vi "VS Async VI_Example.vi"() -> ()   [LabVIEW 2011]
uses:
  CANOpen Addon Custom Device.lvlib
panel:
  in  "stop":bool
  in  "Error":errorcluster
  out "error out":errorcluster
  in  "Parent":string
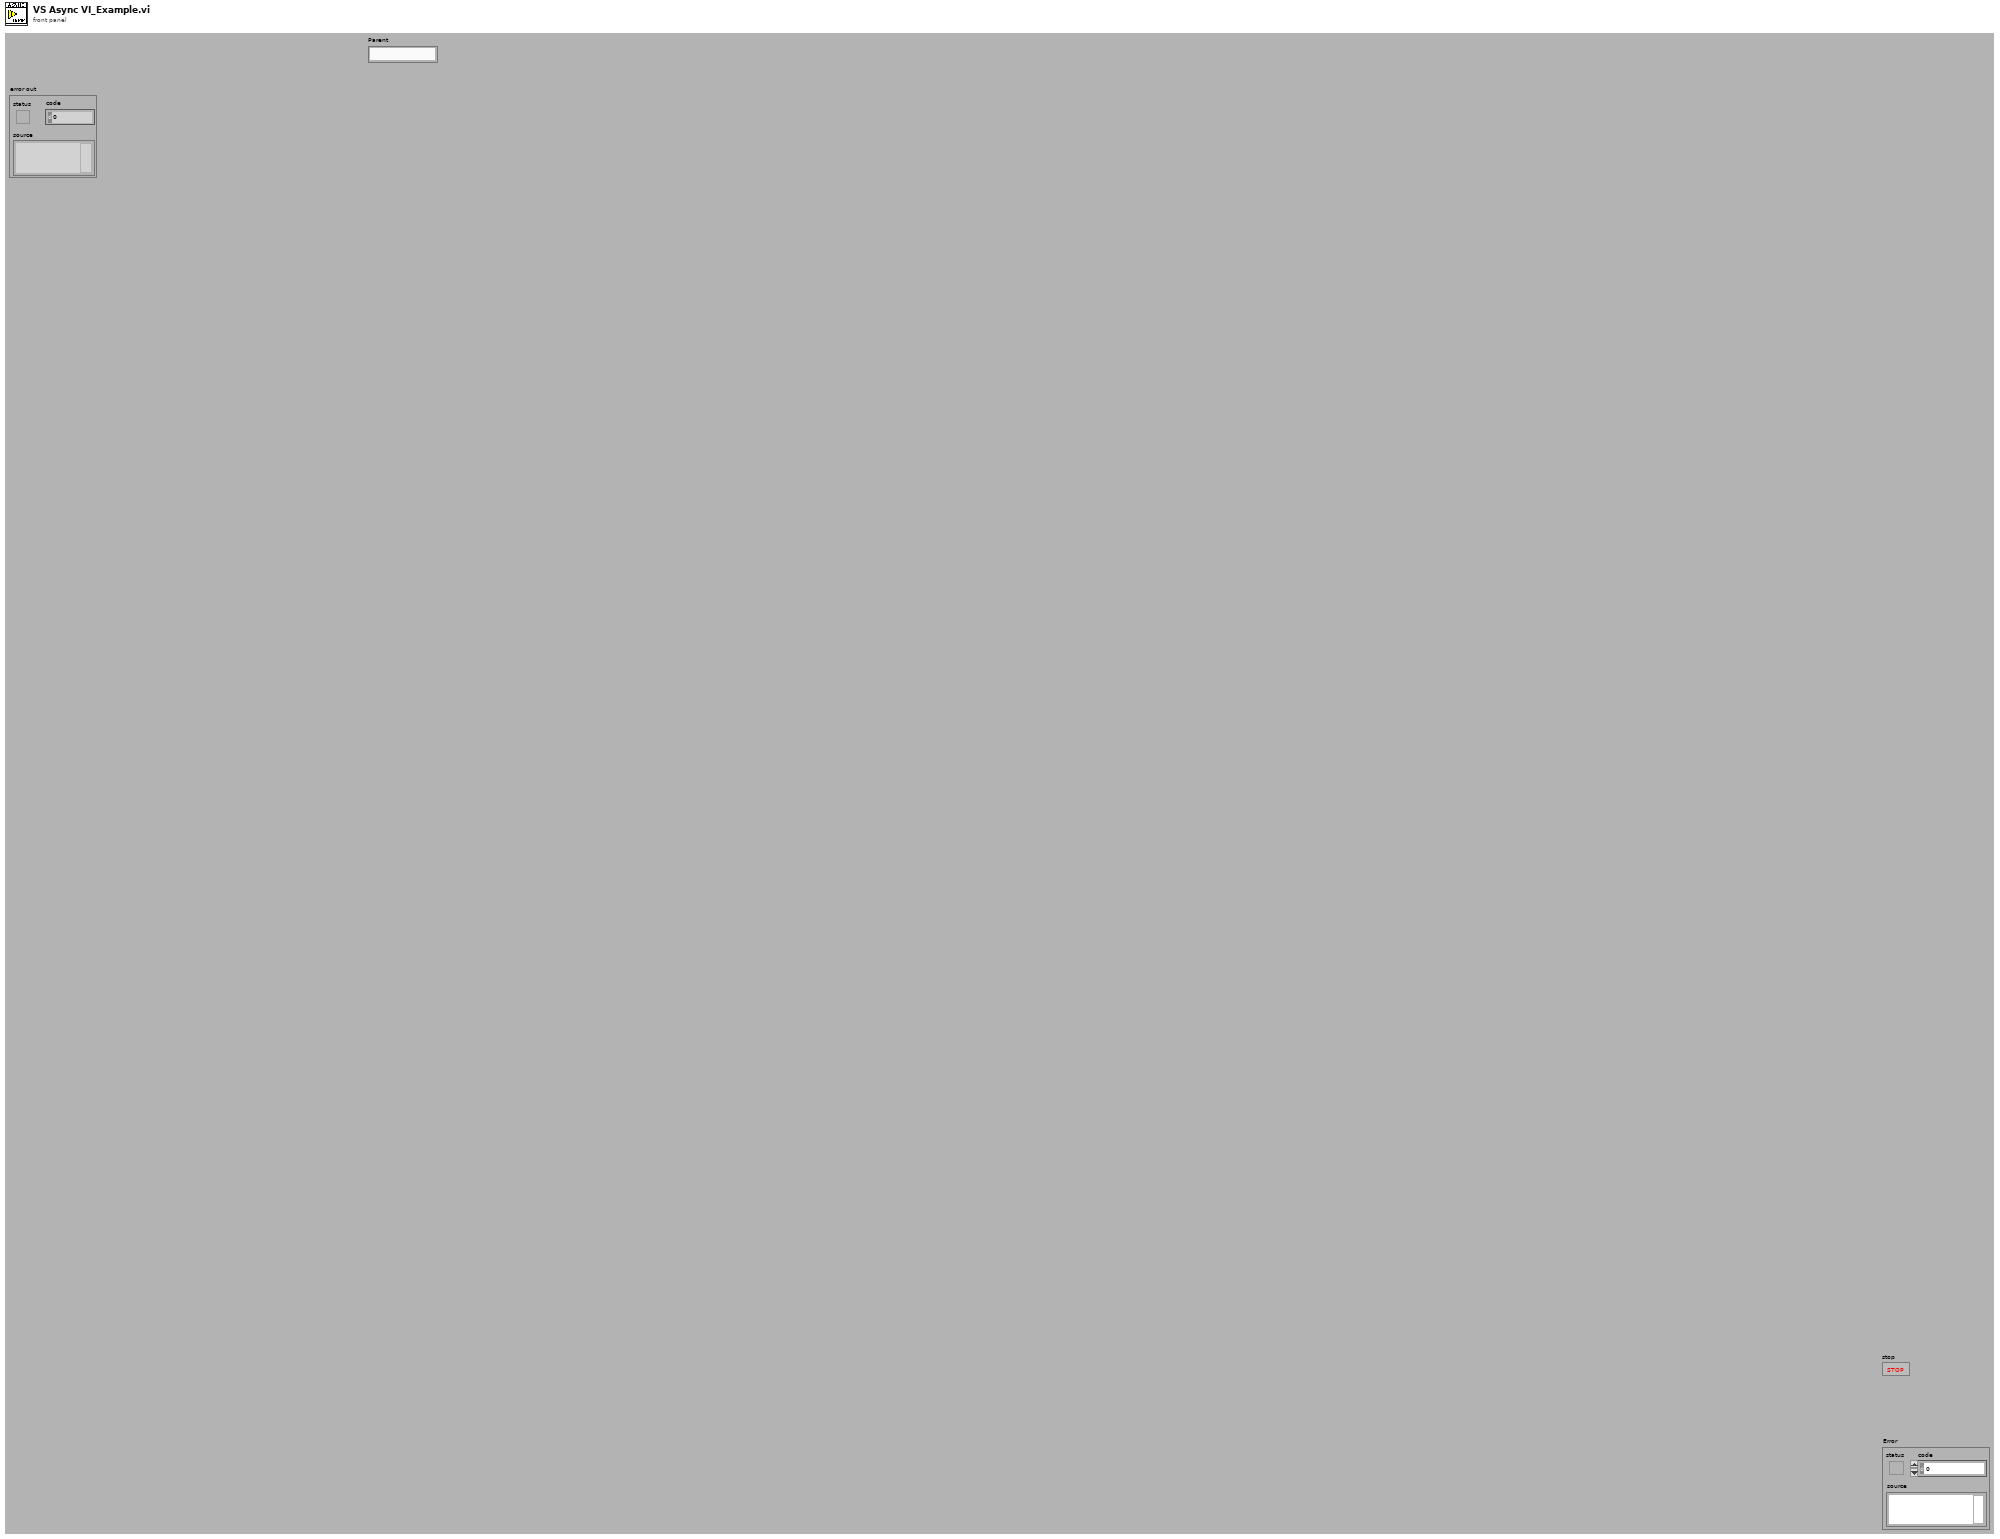
[diagram p1: front panel]
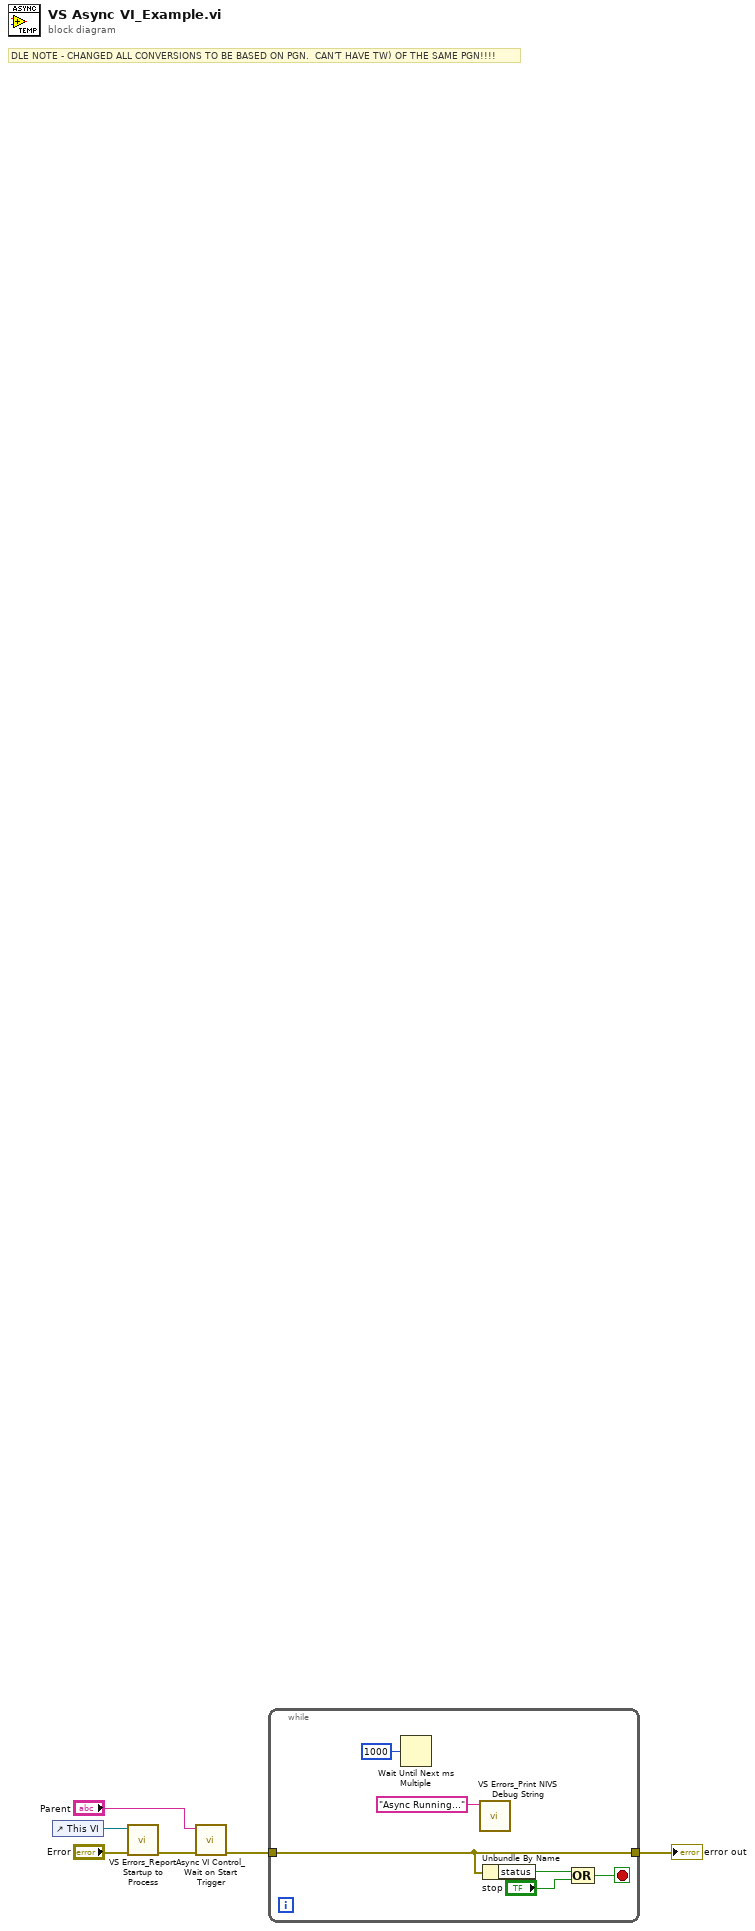
[diagram p0: block diagram]
diagram:
  # "DLE NOTE - CHANGED ALL CONVERSIONS TO BE BASED ON PGN.  CAN'T HAVE TW) OF THE SAME PGN!!!!"
  n1 = control-ref of="This VI"() -> (w5:refnum<vi>)
  n2 = call "VS Errors_Report Startup to Process.vi"("Error"="Error", "This VI"=w5) -> ("error out"=w6:errorcluster)  [unwired: 9 in]
  n3 = call "Async VI Control_Wait on Start Trigger.vi"("error in (no error)"=w6, "Name"="Parent") -> ("error out"=w1:errorcluster)  [unwired: 8 in, 1 out]
  n4 = while {
    tunnel: [w10] -> w2
    tunnel: w1 -> [w10]
    stop <- w7 stop-if-true
    n5 = Wait Until Next ms Multiple(millisecond multiple=u32 1000) -> ()  [unwired: 1 out]
    n6 = call "VS Errors_Print NIVS Debug String.vi"("Debug String"="Async Running...") -> ()  [unwired: 9 in, 1 out]
    n7 = Unbundle By Name(w10) -> ("status"=w9:bool)
    n8 = Compound Arithmetic op=OR(w9, "stop") -> (w7:bool)
  }
  "error out" <- w2
